vi "m1m3_getEvent_HardpointMonitorWarning.vi"(8 "error in (no error)":errorcluster, 11 "logevent_HardpointMonitorWarning_Ctl":T1) -> (0 "error out":errorcluster, 2 "function return":i32, 3 "logevent_HardpointMonitorWarning_Ctl out":T1)   [LabVIEW 2016, in "SALLV_m1m3.lvlib"]
doc: "int m1m3_shm_getEvent_HardpointMonitorWarningLV(m1m3_logevent_HardpointMonitorWarningLV *logevent_HardpointMonitorWarning_Ctl );"
uses:
  SALLV_m1m3.lvlib
  DataTypes/logevent_HardpointMonitorWarning.ctl
  SALLV_m1m3.so
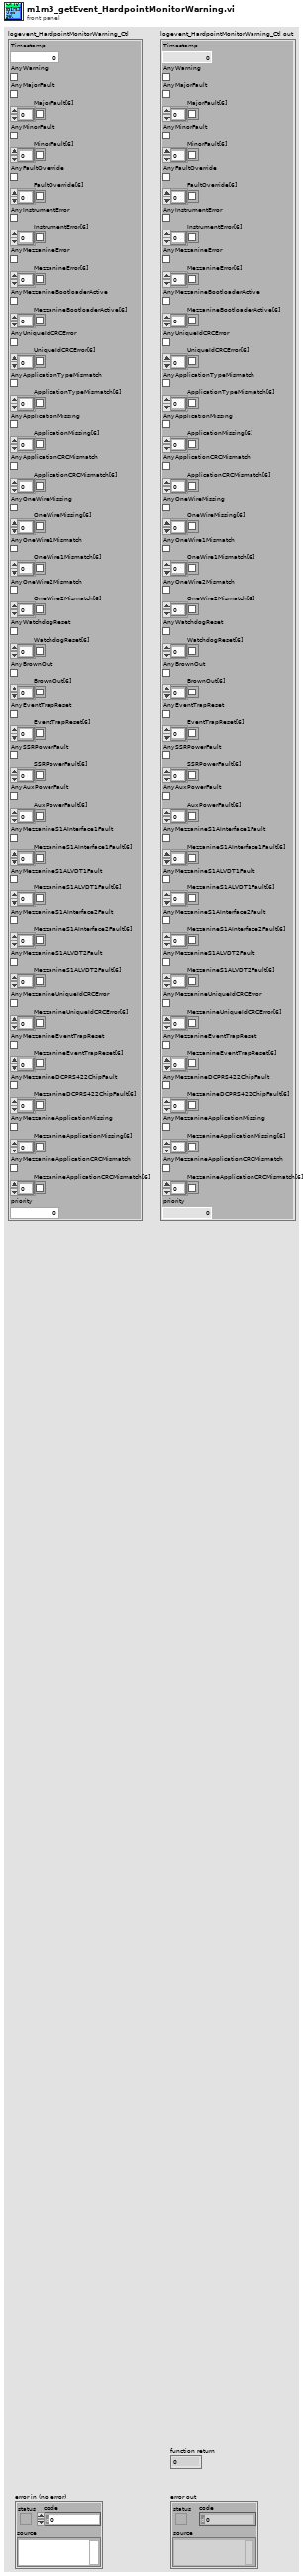
[diagram p1: front panel]
types:
  T1 = typedef "SALLV_m1m3.lvlib/logevent_HardpointMonitorWarning.ctl" = cluster{"Timestamp":dbl, "AnyWarning":bool, "AnyMajorFault":bool, "MajorFault[6]":bool[], "AnyMinorFault":bool, "MinorFault[6]":bool[], "AnyFaultOverride":bool, "FaultOverride[6]":bool[], "AnyInstrumentError":bool, "InstrumentError[6]":bool[], "AnyMezzanineError":bool, "MezzanineError[6]":bool[], "AnyMezzanineBootloaderActive":bool, "MezzanineBootloaderActive[6]":bool[], "AnyUniqueIdCRCError":bool, "UniqueIdCRCError[6]":bool[], "AnyApplicationTypeMismatch":bool, "ApplicationTypeMismatch[6]":bool[], "AnyApplicationMissing":bool, "ApplicationMissing[6]":bool[], "AnyApplicationCRCMismatch":bool, "ApplicationCRCMismatch[6]":bool[], "AnyOneWireMissing":bool, "OneWireMissing[6]":bool[], "AnyOneWire1Mismatch":bool, "OneWire1Mismatch[6]":bool[], "AnyOneWire2Mismatch":bool, "OneWire2Mismatch[6]":bool[], "AnyWatchdogReset":bool, "WatchdogReset[6]":bool[], "AnyBrownOut":bool, "BrownOut[6]":bool[], "AnyEventTrapReset":bool, "EventTrapReset[6]":bool[], "AnySSRPowerFault":bool, "SSRPowerFault[6]":bool[], "AnyAuxPowerFault":bool, "AuxPowerFault[6]":bool[], "AnyMezzanineS1AInterface1Fault":bool, "MezzanineS1AInterface1Fault[6]":bool[], "AnyMezzanineS1ALVDT1Fault":bool, "MezzanineS1ALVDT1Fault[6]":bool[], "AnyMezzanineS1AInterface2Fault":bool, "MezzanineS1AInterface2Fault[6]":bool[], "AnyMezzanineS1ALVDT2Fault":bool, "MezzanineS1ALVDT2Fault[6]":bool[], "AnyMezzanineUniqueIdCRCError":bool, "MezzanineUniqueIdCRCError[6]":bool[], "AnyMezzanineEventTrapReset":bool, "MezzanineEventTrapReset[6]":bool[], "AnyMezzanineDCPRS422ChipFault":bool, "MezzanineDCPRS422ChipFault[6]":bool[], "AnyMezzanineApplicationMissing":bool, "MezzanineApplicationMissing[6]":bool[], "AnyMezzanineApplicationCRCMismatch":bool, "MezzanineApplicationCRCMismatch[6]":bool[], "priority":i32}
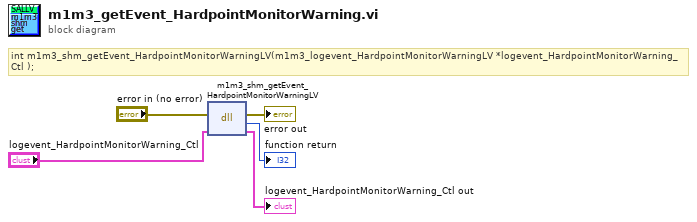
[diagram p0: block diagram]
diagram:
  # "int m1m3_shm_getEvent_HardpointMonitorWarningLV(m1m3_logevent_HardpointMonitorWarningLV *logevent_HardpointMonitorWarning_Ctl );"
  n1 = dll-call lib="opt/CODE/SALLV_m1m3/SALLV_m1m3.*" fn="m1m3_shm_getEvent_HardpointMonitorWarningLV"(error in="error in (no error)", "logevent_HardpointMonitorWarning_Ctl"="logevent_HardpointMonitorWarning_Ctl") -> (error out=→"error out":errorcluster, →"function return":i32, "logevent_HardpointMonitorWarning_Ctl"=→"logevent_HardpointMonitorWarning_Ctl out":T1)  [unwired: 2 in, 1 out]
